vi "Byte Buffer.Write (Boolean).vi"(8 "error in (no error)":errorcluster, 9 "value":bool, 10 "buffer offset":u64, 11 "Byte Buffer in":refnum<class "Byte Buffer.lvclass">) -> (0 "error out":errorcluster, 3 "Byte Buffer out":refnum<class "Byte Buffer.lvclass">)   [LabVIEW 2016, in "VeriStand Data.lvlib" / "Byte Buffer.lvclass"]
doc: "Writes <B>value</B> to the provided <B>Byte Buffer</B> at location <B>buffer offset</B> in the format of the data type specified."
uses:
  Byte Buffer.lvclass
  Byte Buffer.lvclass/Byte Buffer.ctl
  Byte Buffer.Buffer Subset.Set.vi
  Memory Management/Memory Management.MoveByteBlock.Read (String).vi
  Memory Management/Memory Management.Handle Return.vi
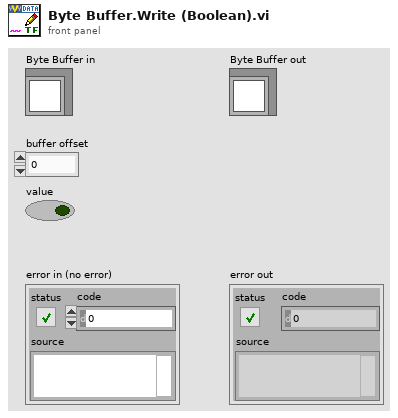
[diagram p1: front panel]
types:
  T1 = enum16{"big-endian, network order", "native, host order", "little-endian"}
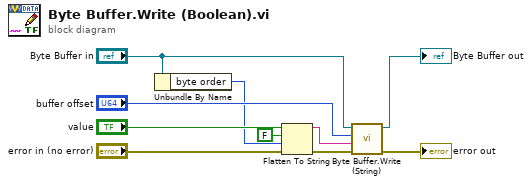
[diagram p0: block diagram]
diagram:
  n1 = Unbundle By Name("Byte Buffer in") -> ("byte order"=w1:T1)
  n2 = Flatten To String(anything="value", prepend array or string size? (T)=FALSE, byte order (0:big-endian, network order)=w1, error in (no error)="error in (no error)") -> (data string=w8:string, error out=w9:errorcluster)  [unwired: 1 out]
  n3 = call "Byte Buffer.Write (String).vi"("error in (no error)"=w9, "string"=w8, "buffer offset"="buffer offset", "Byte Buffer in"="Byte Buffer in") -> ("error out"=→"error out":errorcluster, "Byte Buffer out"=→"Byte Buffer out":refnum<class "Byte Buffer.lvclass">)  [unwired: 6 in]
